vi "Read Modules Configurations.vi"(8 "error in":errorcluster, 11 "Engine Parent in":refnum<class "Engine Parent Editor Node.lvclass">) -> (0 "error out":errorcluster, 2 "Component Configurations":refnum<class "TBM module configuration.lvclass">[](array[class]), 3 "Engine Parent out":refnum<class "Engine Parent Editor Node.lvclass">)   [LabVIEW 2013, in "PL Framework Configuration Tool.lvlib" / "Engine Parent Editor Node.lvclass"]
uses:
  Engine Parent Editor Node.lvclass
  <vilib>/NI/Tag Bus Module Framework/module configuration/TBM module configuration.lvclass
  <vilib>/CEF_TreeControl/Node/NISE_CEF_Node.lvclass/NISE_CEF_Node.ctl
  Module editor node/module editor node.lvclass
  asynchronous execution module/configuration/asynchronous execution module configuration.lvclass
  asynchronous execution module/configuration/asynchronous execution module configuration.lvclass/asynchronous execution module configuration.ctl
  <vilib>/CEF_TreeControl/Node/NISE_CEF_Node.lvclass
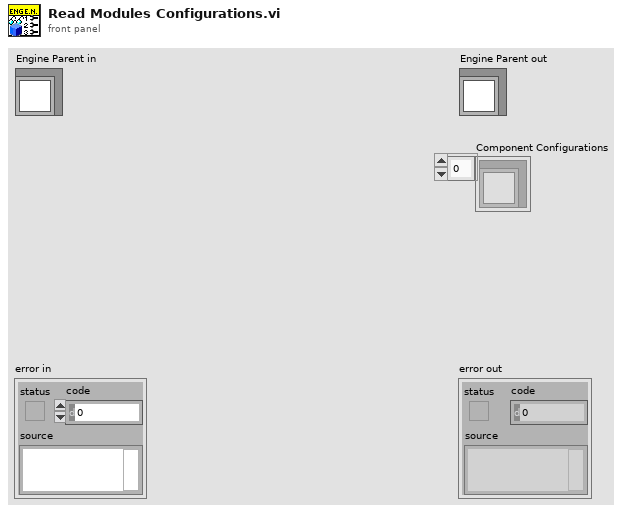
[diagram p1: front panel]
types:
  T1 = typedef "NISE_CEF_Node.lvclass/NodeRef.ctl" = refnum<data-value>
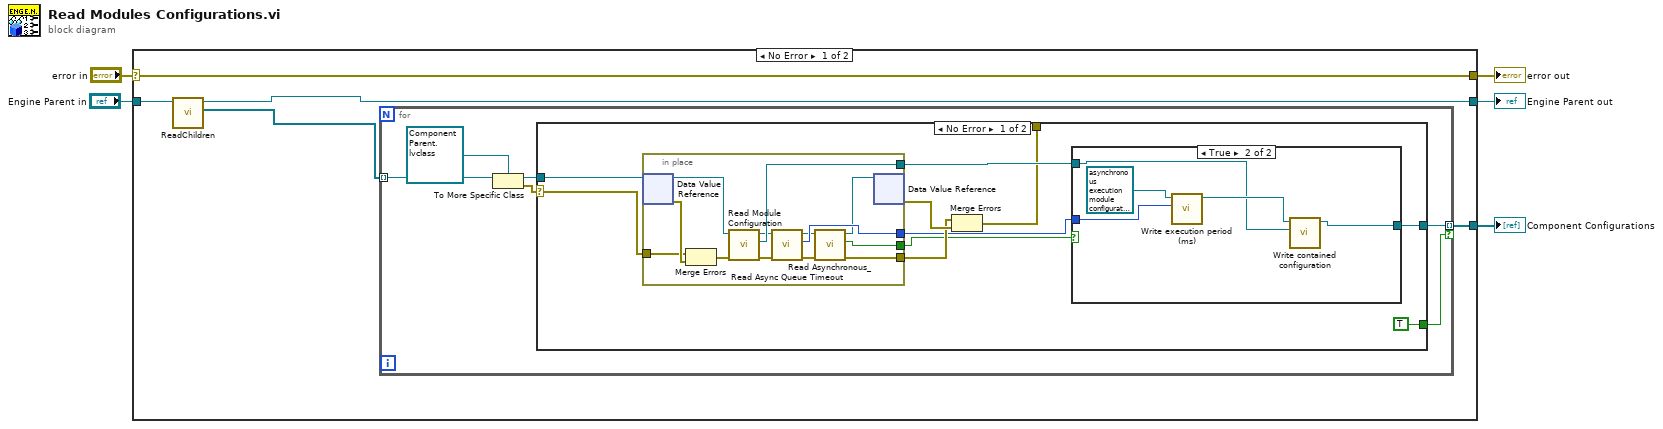
[diagram p0: block diagram]
diagram:
  n1 = case shown="No Error" "error in" {
    selector: "error in" -> [w10 w46]
    tunnel: [w10 w46] -> w4
    tunnel: [w7 w47] -> w2
    tunnel: "Engine Parent in" -> [w8 w47]
    tunnel: [w9 _] -> w1
    frame No Error {
      n2 = call <vilib>:"ReadChildren.vi"("node in"=w8) -> ("output array"=w6:T1[], "node out"=w7:refnum<class "Engine Parent Editor Node.lvclass">)  [unwired: 8 in, 1 out]
      n3 = for {
        tunnel: w6 -> [w16] mode=indexing
        tunnel: [w13] -> w9 mode=indexing if=w11
        n4 = To More Specific Class(target class=refnum<data-value> refnum ("data value reference"), reference=w16) -> (specific class reference=w14:refnum<data-value>, error out=w12:errorcluster)  [unwired: 1 in]
        n5 = case shown="No Error" w12 {
          selector: w12 -> [w22 _]
          tunnel: w14 -> [w21 _]
          tunnel: [w25 _] -> w13
          tunnel: [TRUE _] -> w11
          tunnel: [w19 _] -> _
          frame No Error {
            n6 = in-place {
              in-place-border: [w27] -> w23
              in-place-border: [w38] -> w20
              in-place-border: w22 -> [w30]
              in-place-border: [w37] -> w18
              in-place-border: [w36] -> w17
              n7 = in-place-dvr #1(w21) -> (w39:refnum<class "module editor node.lvclass">, w31:errorcluster)
              n8 = Merge Errors(w30, w31) -> (w29:errorcluster)
              n9 = call "Read Module Configuration.vi"("error in"=w29, "Module Editor Node in"=w39) -> ("error out"=w32:errorcluster, "module configuration"=w38:refnum<class "TBM module configuration.lvclass">, "Module Editor Node out"=w33:refnum<class "module editor node.lvclass">)  [unwired: 7 in]
              n10 = call-dynamic "Read Async Queue Timeout.vi"("error in"=w32, "Module Editor Node in"=w33) -> ("error out"=w28:errorcluster, "Queue Timeout"=w36:i32, "Module Editor Node out"=w34:refnum<class "module editor node.lvclass">)  [unwired: 7 in]
              n11 = call-dynamic "Read Asynchronous_.vi"("error in"=w28, "Module Editor Node in"=w34) -> ("error out"=w27:errorcluster, "Asynchronous?"=w37:bool, "Module Editor Node out"=w35:refnum<class "module editor node.lvclass">)  [unwired: 7 in]
              n12 = in-place-dvr #1(w35) -> (w24:errorcluster)  [unwired: 1 out]
            }
            n13 = Merge Errors(w23, w24) -> (w19:errorcluster)
            n14 = case shown="True" w18 {
              tunnel: [w40 w41] -> w25
              tunnel: w17 -> [_ w44]
              tunnel: w20 -> [w40 w42]
              frame False {
              }
              frame True {
                n15 = call "Write execution period (ms).vi"("execution period (ms)"=w44, "Asynchronous Component Configuration in"=refnum<class "asynchronous execution module configuration.lvclass"> refnum ("Asynchronous Component Configuration")) -> ("Asynchronous Component Configuration out"=w43:refnum<class "asynchronous execution module configuration.lvclass">)  [unwired: 8 in, 1 out]
                n16 = call "Write contained configuration.vi"("module configuration"=w42, "asynchronous execution module configuration in"=w43) -> ("asynchronous execution module configuration out"=w41:refnum<class "asynchronous execution module configuration.lvclass">)  [unwired: 8 in, 1 out]
              }
            }
          }
          frame Error {
          }
        }
      }
    }
    frame Error {
    }
  }
  "error out" <- w4
  "Engine Parent out" <- w2
  "Component Configurations" <- w1
